vi "item select mouse down action.vi"(8 "error in (no error)":errorcluster, 10 "Mouse down data":T1, 11 "Loop data":T2) -> (0 "error out":errorcluster, 2 "New Selection states":bool[](array[boolean]), 3 "Loop data":T2)   [LabVIEW 2020, in "UI_ItemSelect.lvlib"]
uses:
  UI_ItemSelect.lvlib
  Tree item select loop data.ctl
  Item select ref type.ctl
  Tree item loop data.ctl
  Tree item selection indices.ctl
  checkbox state.ctl
  item select tree lock states.ctl
  item select mouse down data.ctl
  item select calc action.ctl
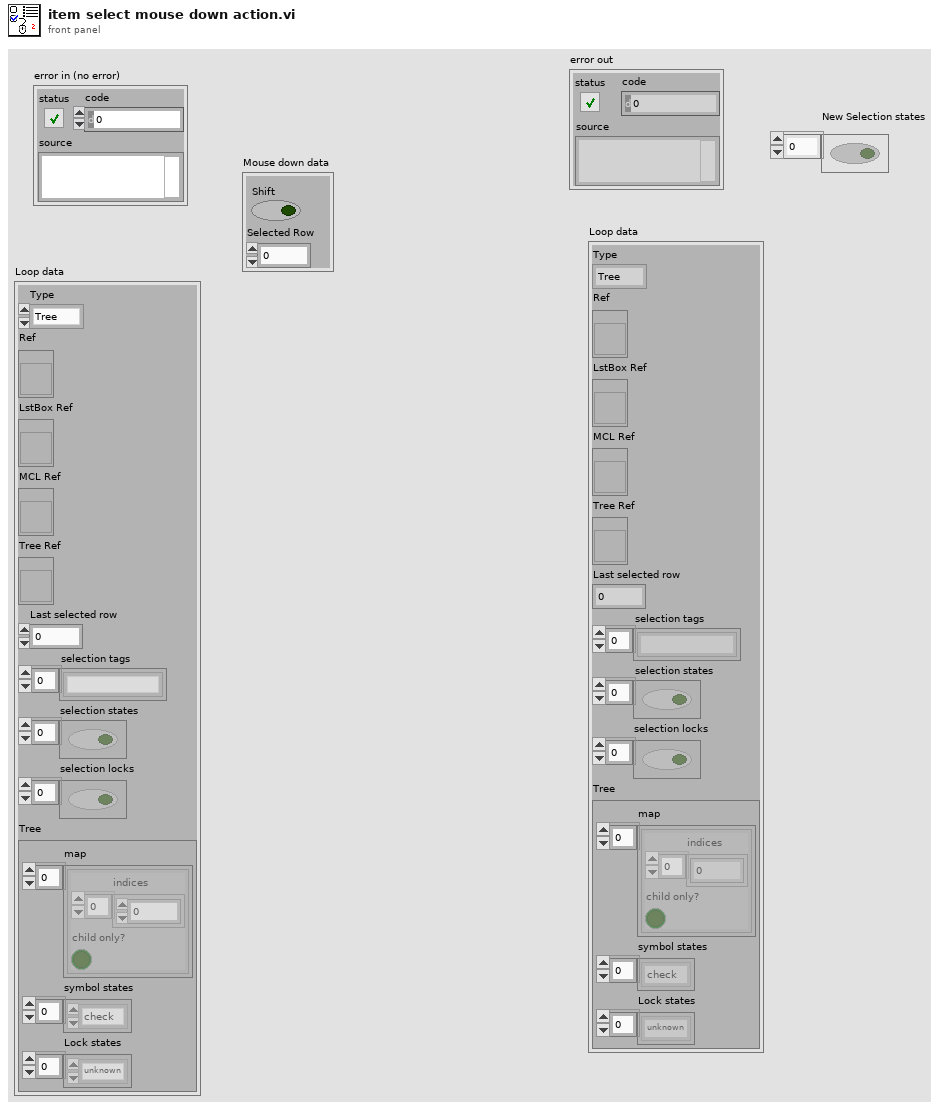
[diagram p1: front panel]
types:
  T1 = typedef "UI_ItemSelect.lvlib/item select mouse down data.ctl" = cluster{"Shift":bool, "Selected Row":i32}
  T2 = typedef "UI_ItemSelect.lvlib/Tree item select loop data.ctl" = cluster{"Type":T3, "Ref":refnum<vi>, "LstBox Ref":refnum<vi>, "MCL Ref":refnum<vi>, "Tree Ref":refnum<vi>, "Last selected row":i32, "selection tags":string[], "selection states":bool[], "selection locks":bool[], "Tree":T4}
  T3 = typedef "UI_ItemSelect.lvlib/Item select ref type.ctl" = enum16{"Tree", "MCL", "ListBox"}
  T4 = typedef "UI_ItemSelect.lvlib/Tree item loop data.ctl" = cluster{"map":T5[], "symbol states":T6[], "Lock states":T7[]}
  T5 = typedef "UI_ItemSelect.lvlib/Tree item selection indices.ctl" = cluster{"indices":i32[], "child only?":bool}
  T6 = typedef "UI_ItemSelect.lvlib/checkbox state.ctl" = enum16{"unknown", "check", "some", "no check"}
  T7 = typedef "UI_ItemSelect.lvlib/item select tree lock states.ctl" = enum16{"unknown", "locked", "unlocked"}
  T8 = typedef "UI_ItemSelect.lvlib/item select calc action.ctl" = enum16{"false", "true", "invert"}
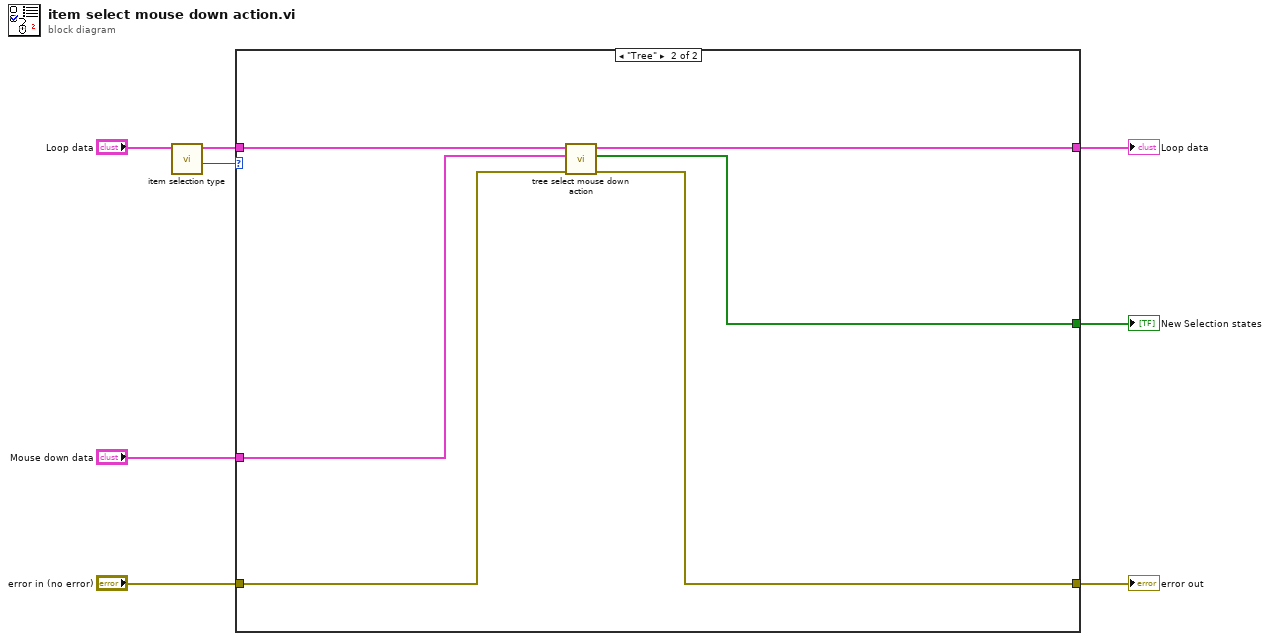
[diagram p0: block diagram]
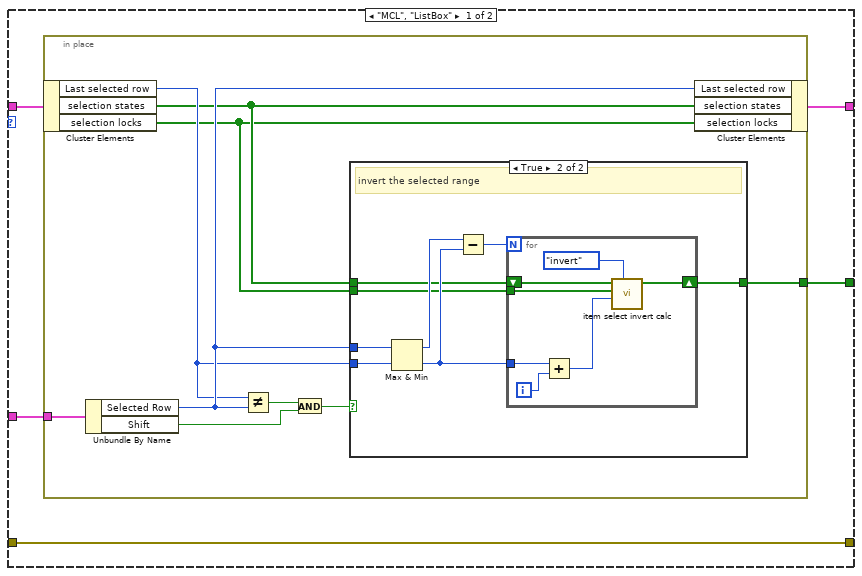
[diagram p2: hidden frame]
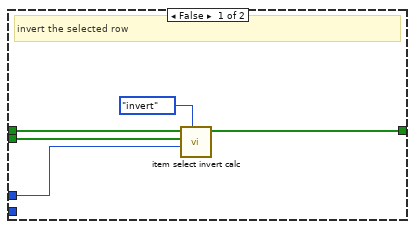
[diagram p3: hidden frame]
diagram:
  n1 = call "item selection type.vi"("Loop data"="Loop data") -> ("Type"=w7:T3, "Loop data"=w6:T2)  [unwired: 9 in]
  n2 = case shown="\"Tree\"" w7 {
    tunnel: w6 -> [w13 w48]
    tunnel: "error in (no error)" -> [w9 w47]
    tunnel: [w9 w46] -> w4
    tunnel: [w11 w45] -> w3
    tunnel: [w10 w44] -> w2
    tunnel: "Mouse down data" -> [w12 w43]
    frame "MCL", "ListBox" {
      n3 = in-place {
        in-place-border: w12 -> [w20]
        in-place-border: [w14] -> w10
        n4 = in-place-cluster #1(w13) -> ("Last selected row"=w17:i32, "selection states"=w16:bool[], "selection locks"=w15:bool[])
        n5 = Unbundle By Name(w20) -> ("Selected Row"=w18:i32, "Shift"=w21:bool)
        n6 = Not Equal?(x=w17, y=w18) -> (x != y?=w22:bool)
        n7 = And(x=w22, y=w21) -> (x .and. y?=w19:bool)
        n8 = case shown="True" w19 {
          tunnel: w18 -> [w25 w35]
          tunnel: w17 -> [_ w34]
          tunnel: w16 -> [w27 w30]
          tunnel: w15 -> [w26 w29]
          tunnel: [w24 w28] -> w14
          frame False {
            # "invert the selected row"
            n9 = call "item select invert calc.vi"("Action"=item_select_calc_action."invert", "selection index"=w25, "selection locks"=w26, "selection states"=w27) -> ("new selection states"=w24:bool[])  [unwired: 7 in]
          }
          frame True {
            # "invert the selected range"
            n10 = Max & Min(x=w35, y=w34) -> (max(x,y)=w33:i32, min(x,y)=w31:i32)
            n11 = Subtract(x=w33, y=w31) -> (x-y=w32:i32)
            n12 = for {
              N: w32 -> [_]
              tunnel: w31 -> [w42]
              shift-right: [w39] -> w28
              shift-left: w30 -> [w40]
              tunnel: w29 -> [w37]
              i -> [w41]
              n13 = Add(x=w42, y=w41) -> (x+y=w38:i32)
              n14 = call "item select invert calc.vi"("Action"=item_select_calc_action."invert", "selection index"=w38, "selection locks"=w37, "selection states"=w40) -> ("new selection states"=w39:bool[])  [unwired: 7 in]
            }
          }
        }
        n15 = in-place-cluster #1("Last selected row"=w18, "selection states"=w16, "selection locks"=w15) -> (w11:T2)
      }
    }
    frame "Tree" {
      n16 = call "tree select mouse down action.vi"("error in (no error)"=w47, "Mouse down data"=w43, "Loop data"=w48) -> ("error out"=w46:errorcluster, "New Selection states"=w44:bool[], "Loop data"=w45:T2)  [unwired: 6 in]
    }
  }
  "Loop data" <- w3
  "error out" <- w4
  "New Selection states" <- w2
